vi "ma_FFT with Hanning.vi"(4 "exclude Nyquist":bool=TRUE, 6 "correct DC":bool=TRUE, 11 "time signal data":dbl[](array[numeric])) -> (2 "FFT size":i32, 3 "complex Hann spectrum":cdb[](array[numeric]))   [LabVIEW 2020, in "NI_MAPro.lvlib"]
uses:
  NI_MAPro.lvlib
  NI_AALPro.lvlib
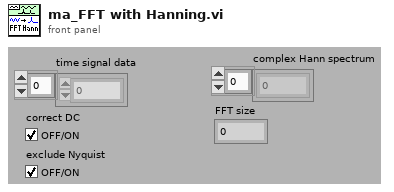
[diagram p1: front panel]
types:
  T1 = enum16{"Rectangular (none)", "Hanning", "Low side lobe"}
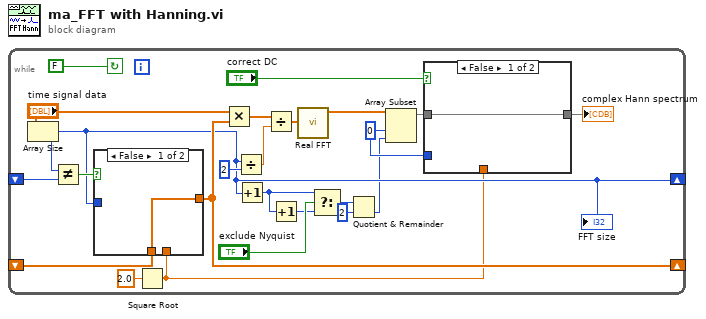
[diagram p0: block diagram]
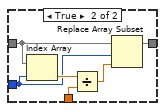
[diagram p2: hidden frame]
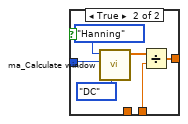
[diagram p3: hidden frame]
diagram:
  n1 = while {
    shift-left: _ -> [w18]
    shift-right: [w17] -> _
    shift-left: _ -> [w16]
    shift-right: [w14] -> _
    stop <- FALSE continue-if-true
    w9 = 0
    n2 = Array Size(array="time signal data") -> (size(s)=w14:i32)
    "FFT size" <- w14
    n3 = Not Equal?(x=w14, y=w16) -> (x != y?=w15:bool)
    n4 = Square Root(x=2.0) -> (sqrt(x)=w10:dbl)
    n5 = case shown="False" w15 {
      tunnel: w14 -> [_ w38]
      tunnel: [w32 w34] -> w17
      tunnel: w18 -> [w32 _]
      tunnel: w10 -> [_ w33]
      frame False {
      }
      frame True {
        n6 = call "ma_Calculate window.vi"("scaled for"=enum16{"DC", "RMS"}."DC", "array size"=w38, "window"=T1."Hanning") -> ("Window data"=w35:dbl[])  [unwired: 8 out]
        n7 = Divide(x=w35, y=w33) -> (x/y=w34:dbl[])
      }
    }
    n8 = Multiply(x="time signal data", y=w17) -> (x*y=w19:dbl[])
    n9 = Divide(x=w14, y=2) -> (x/y=w22:dbl)
    n10 = Increment(x=w14) -> (x+1=w1:i32)
    n11 = Divide(x=w19, y=w22) -> (x/y=w24:dbl[])
    n12 = Increment(x=w1) -> (x+1=w2:i32)
    n13 = call "Real FFT.vi"("X"=w24) -> ("FFT {X}"=w21:cdb[])  [unwired: 9 in, 1 out]
    n14 = Select(t=w1, s="exclude Nyquist", f=w2) -> (s? t:f=w3:i32)
    n15 = Quotient & Remainder(x=w3, y=2) -> (floor(x/y)=w4:i32)  [unwired: 1 out]
    n16 = Array Subset(array=w21, index=w9, length=w4) -> (w8:cdb[])
    n17 = case shown="False" "correct DC" {
      tunnel: w10 -> [_ w30]
      tunnel: w9 -> [_ w28]
      tunnel: w8 -> [w25 w27]
      tunnel: [w25 w26] -> w7
      frame False {
      }
      frame True {
        n18 = Index Array(array=w27, index=w28) -> (element=w31:cdb)
        n19 = Divide(x=w31, y=w30) -> (x/y=w29:cdb)
        n20 = Replace Array Subset(array=w27, new element=w29, index=w28) -> (w26:cdb[])
      }
    }
    "complex Hann spectrum" <- w7
  }
